vi "Save Editor Position.vi"(8 "error in":errorcluster, 11 "IE VI Ref":refnum<vi>) -> (0 "error out":errorcluster)   [LabVIEW 2021, in "lv_icon.lvlib"]
doc: "Writes the position data to the LabVIEW INI file."
uses:
  <vilib>/LabVIEW Icon API/lv_icon/lv_icon.lvlib
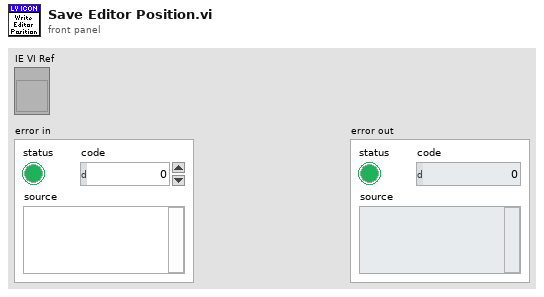
[diagram p1: front panel]
types:
  T1 = typedef "LVRectTypeDef.ctl" = cluster{"Left":i16, "Top":i16, "Right":i16, "Bottom":i16}
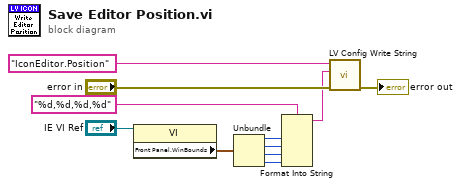
[diagram p0: block diagram]
diagram:
  n1 = property class="VI"(reference="IE VI Ref") -> ("Front Panel.WinBounds"=w9:T1)  [unwired: 1 in, 2 out]
  n2 = Unbundle(w9) -> ("Left"=w8:i16, "Top"=w7:i16, "Right"=w6:i16, "Bottom"=w5:i16)
  n3 = Format Into String(format string="%d,%d,%d,%d", w8, w7, w6, w5) -> (resulting string=w3:string)  [unwired: 2 in, 1 out]
  n4 = call <resource>:"LV Config Write String.vi"("error in (no error)"="error in", "value"=w3, "key"="IconEditor.Position") -> ("error out"=→"error out":errorcluster)  [unwired: 4 in]
